vi "Teleop.vi"(10 "Match Info":T1={"Autonomous Elapsed Seconds"=0.0, "TeleOp Elapsed Seconds"=0.0, "Disabled Elapsed Seconds"=0.0, "Visited Autonomous"=FALSE, "Visited TeleOp"=FALSE, "Visited Disabled"=FALSE, "Autonomous Settings"={"Autonomous Style"=enum."Independent", "VI Refnum"=refnum}}, 11 "Call Context":T2) -> ()   [LabVIEW 2015]
doc: "This VI is called for each TeleOp packet received from the DS where the robot is not disabled. It is often used to read from the joysticks and update I/O or to update setpoints for timed control loops. It should complete and return within 20 milliseconds or it may miss DS packets."
uses:
  <vilib>/Rock Robotics/WPI/DriverStation/WPI_DriverStationDerivedRobotMode.ctl
  <vilib>/Rock Robotics/WPI/DriverStation/WPI_DriverStationMatch Info.ctl
  Robot Global Data.vi
  <vilib>/Rock Robotics/Network Tables/SD Write Number.vi
  <vilib>/Rock Robotics/WPI/Solenoid/Deprecated/WPI_SolenoidSetBool.vi
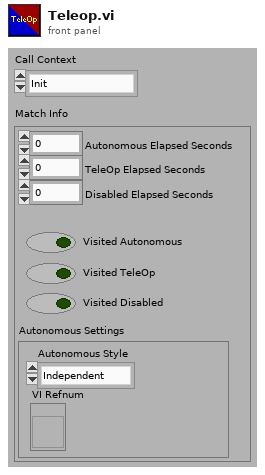
[diagram p1: front panel]
types:
  T1 = typedef "WPI_DriverStationMatch Info.ctl" = cluster{"Autonomous Elapsed Seconds":dbl, "TeleOp Elapsed Seconds":dbl, "Disabled Elapsed Seconds":dbl, "Visited Autonomous":bool, "Visited TeleOp":bool, "Visited Disabled":bool, "Autonomous Settings":cluster{"Autonomous Style":enum16{"Iterative", "Independent"}, "VI Refnum":refnum<vi>}}
  T2 = typedef "WPI_DriverStationDerivedRobotMode.ctl" = enum16{"Init", "Execute", "Stop"}
  T3 = typedef "WPI_MotorControlDeviceRef.ctl" = cluster{"DeviceStatus":errorcluster, "Type":T4, "PWM":cluster{"PWM Channel":T5, "DeadBand":T6}, "CAN":cluster{"Device Number":u8, "Control Mode":T7, "Semaphore":T8, "Max Vout":dbl, "TalonSRX Control Mode":T9}, "Invert":bool}
  T4 = typedef "WPI_MotorControlType.ctl" = enum16{"PWM", "CAN", "CANTalonSRX"}
  T5 = typedef "FPGA_DIOPWMChannel.ctl" = enum8{"PWM 0", "PWM 1", "PWM 2", "PWM 3", "PWM 4", "PWM 5", "PWM 6", "PWM 7", "PWM 8", "PWM 9", "PWM MXP 0", "PWM MXP 1", "PWM MXP 2", "PWM MXP 3", "PWM MXP 4", "PWM MXP 5", "PWM MXP 6", "PWM MXP 7", "PWM MXP 8", "PWM MXP 9", "Invalid"}
  T6 = typedef "WPI_PWMDeadband.ctl" = cluster{"Name":string, "maxPositivePwm":i32, "minPositivePwm":i32, "centerPwm":i32, "maxNegativePwm":i32, "minNegativePwm":i32, "angularRange":u16}
  T7 = typedef "WPI_CANJaguar_ControlMode.ctl" = enum8{"Percent VBus", "Current", "Speed", "Position", "Voltage"}
  T8 = typedef "Semaphore RefNum" = refnum<k1>
  T9 = typedef "WPI_CANTalonSRX_APIControlMode.ctl" = enum8{"Percent VBus", "Speed", "Position", "Slave", "Unchanged / Invalid", "Voltage Compensation", "Current", "Motion Profile"}
  T10 = typedef "WPI_CANTalonSRX_GlobalStatus.ctl" = cluster{"Applied Throttle":dbl, "Module Enabled":bool, "CAN Error":errorcluster, "Closed Loop Error":dbl, "Forward Limit Switch Closed":bool, "Reverse Limit Switch Closed":bool, "Sensor Position":dbl, "Sensor Velocity":dbl, "Current":dbl, "Sticky Fault - Over Temp":bool, "Sticky Fault - Under Voltage":bool, "Sticky Fault - Forward Limit":bool, "Sticky Fault - Reverse Limit":bool, "Sticky Fault - Forward Soft Limit":bool, "Sticky Fault - Reverse Soft Limit":bool, "Brake is Enabled":bool, "Encoder Position":dbl, "Encoder Velocity":dbl, "Encoder Index Count":dbl, "Encoder A Pin State":bool, "Encoder B Pin State":bool, "Encoder Index Pin State":bool, "Analog In":dbl, "Analog In Velocity":dbl, "Temperature (C)":dbl, "Battery Voltage":dbl, "Control 5 Is Supported":bool, "Current Profile Slot Select":dbl, "Pos Div 8":bool, "Vel Div 4":bool, "Pulse Width Position":i32, "Pulse Width Velocity":i32, "Pulse Width Rise To Rise (us)":i32, "Pulse Width Rise To Fall (us)":i32, "Mot Prof Active Is Under Run":bool, "Mot Prof Active Has Under Run":bool, "Mot Prof Active Is Last":bool, "Mot Prof Active Velocity Only":bool, "Mot Prof Active Is Valid":bool, "Mot Prof Buffer Is Full":bool, "Mot Prof Active Profile Slot Select":i32, "Mot Prof NextID":i32, "Mot Prof Count":i32, "Mot Prof Active Velocity":dbl, "Mot Prof Active Position":dbl, "Mot Prof Output Enable":i32}
  T11 = typedef "WPI_SolenoidDevRef.ctl" = cluster{"DevStatus":errorcluster, "Pneumatics Control Module":u8, "Forward Solenoid Channel":T12, "Reverse Solenoid Channel":T12}
  T12 = typedef "WPI_SolenoidChannel.ctl" = enum8{"Solenoid 0", "Solenoid 1", "Solenoid 2", "Solenoid 3", "Solenoid 4", "Solenoid 5", "Solenoid 6", "Solenoid 7", "Invalid"}
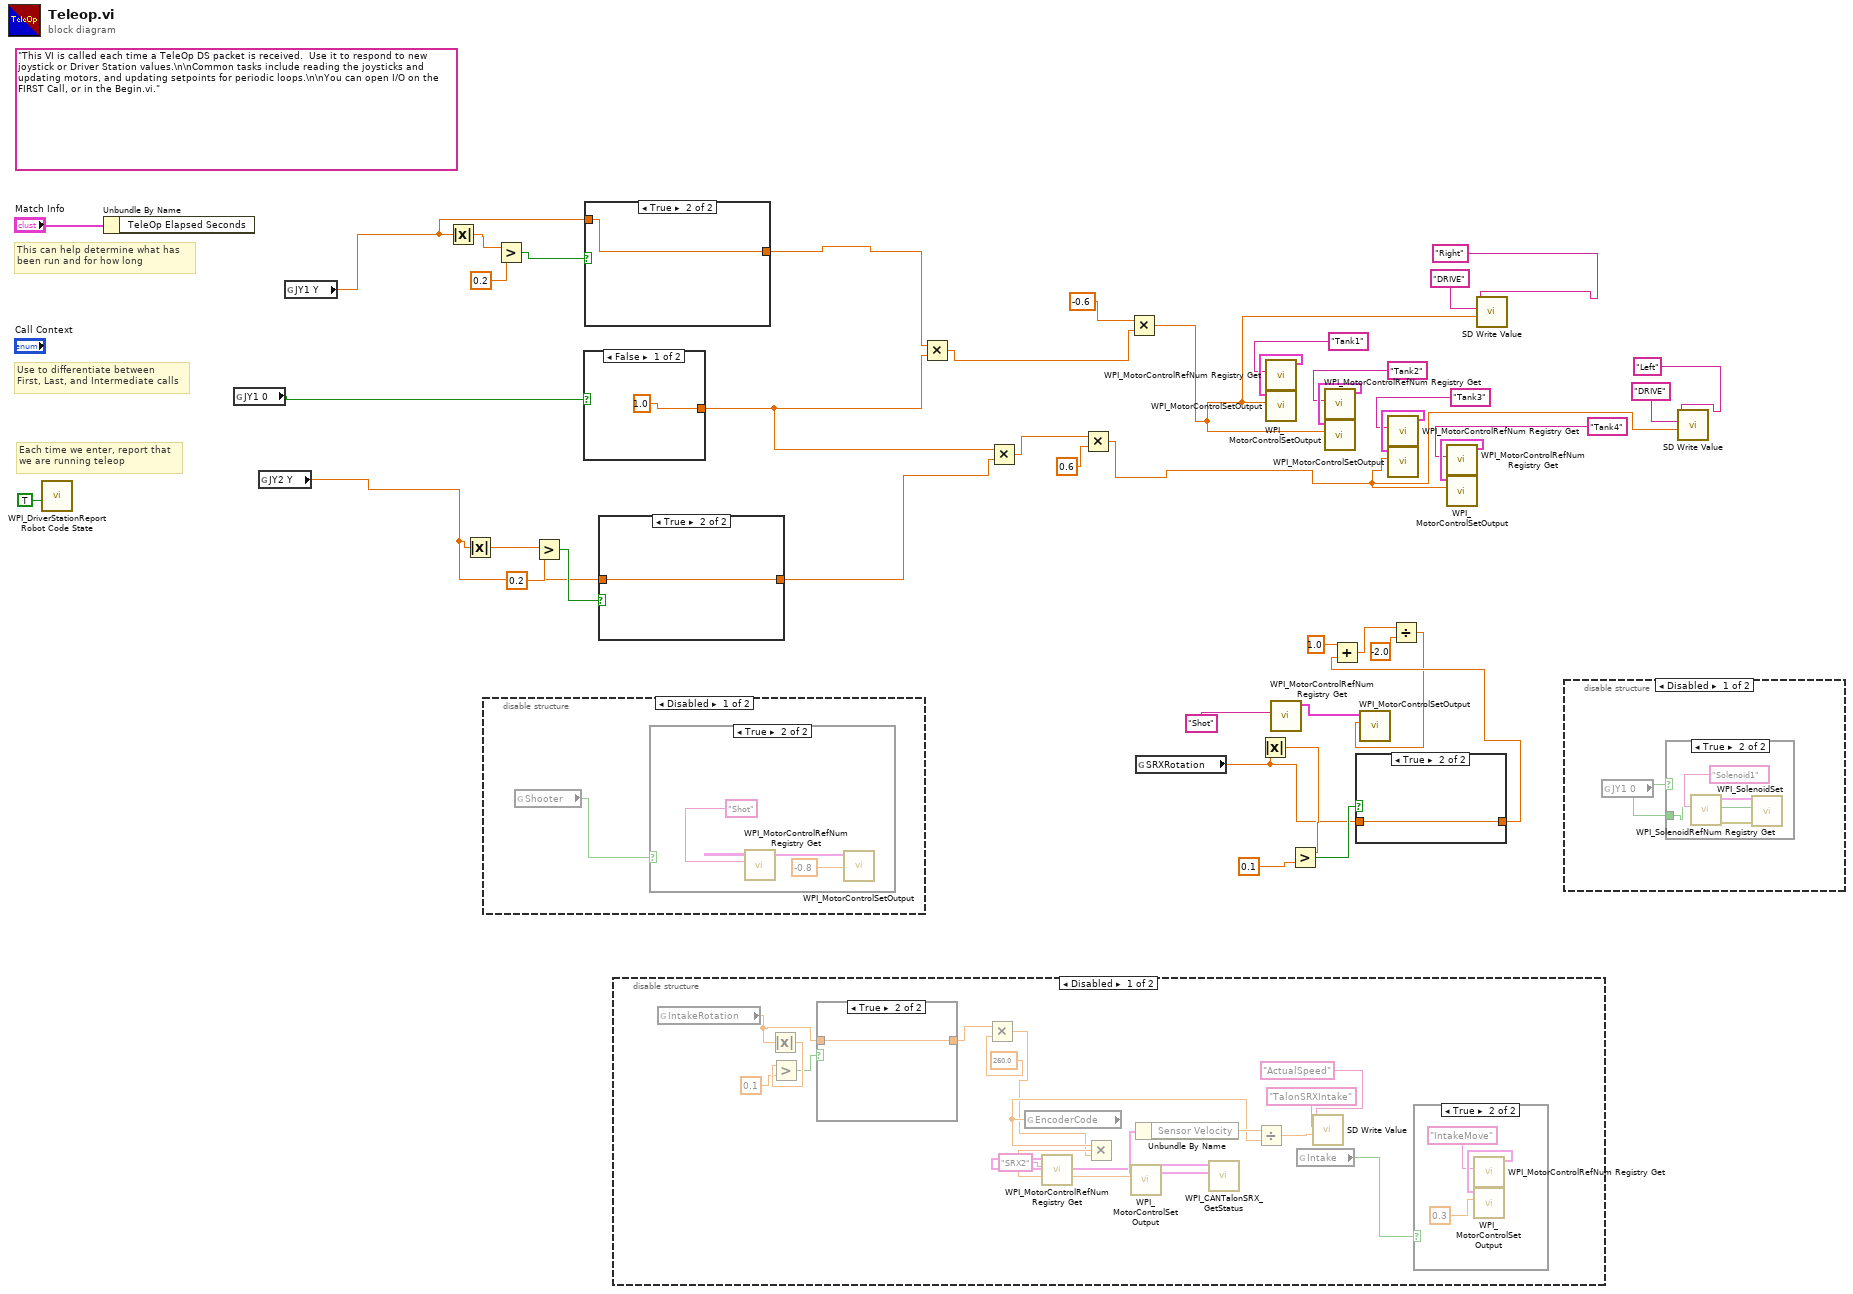
[diagram p0: block diagram]
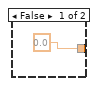
[diagram p6: hidden frame]
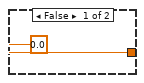
[diagram p9: hidden frame]
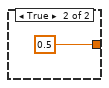
[diagram p10: hidden frame]
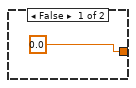
[diagram p11: hidden frame]
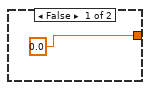
[diagram p12: hidden frame]
diagram:
  (unwired) "This VI is called each time a TeleOp DS packet is received.  Use it to respond to new joystick or Driver Station values.\n\nCommon tasks include reading the joysticks and updating motors, and updating setpoints for periodic loops.\n\nYou can open I/O on the FIRST Call, or in the Begin.vi."
  # "Each time we enter, report that\nwe are running teleop"
  # "Use to differentiate between\nFirst, Last, and Intermediate calls"
  # "This can help determine what has\nbeen run and for how long"
  n1 = call <vilib>:"WPI_DriverStationReport Robot Code State.vi"("TeleOp"=TRUE ("Autonomous")) -> ()  [unwired: 10 in, 1 out]
  n2 = Unbundle By Name("Match Info") -> ()  [unwired: 1 out]
  n3 = global read "Robot Global Data.vi" "JY1 0"() -> (w29:bool)
  n4 = global read "Robot Global Data.vi" "JY2 Y"() -> (w30:dbl)
  n5 = global read "Robot Global Data.vi" "JY1 Y"() -> (w31:dbl)
  n6 = Absolute Value(x=w31) -> (abs(x)=w34:dbl)
  n7 = Absolute Value(x=w30) -> (abs(x)=w33:dbl)
  n8 = disable-structure shown="Disabled" {
    frame Disabled {
      n9 = global read "Robot Global Data.vi" "Shooter"() -> (w44:bool)
      n10 = case shown="True" w44 {
        frame False {
        }
        frame True {
          n11 = call <vilib>:"WPI_MotorControlRefNum Registry Get.vi"("refnum name"="Shot") -> ("MotorControlDevRef"=w47:T3)  [unwired: 9 in, 1 out]
          n12 = call <vilib>:"WPI_MotorControlSetOutput.vi"("Output"=-0.8, "MotorControlDevRef"=w47) -> ()  [unwired: 7 in, 3 out]
        }
      }
    }
    frame Enabled {
    }
  }
  n13 = Greater?(x=w34, y=0.2) -> (0:w41:bool)
  n14 = Greater?(x=w33, y=0.2) -> (0:w39:bool)
  n15 = case shown="False" w29 {
    tunnel: [1.0 0.5] -> w37
    frame False {
    }
    frame True {
    }
  }
  n16 = case shown="True" w41 {
    tunnel: [0.0 w51] -> w13
    tunnel: w31 -> [_ w51]
    frame False {
    }
    frame True {
    }
  }
  n17 = case shown="True" w39 {
    tunnel: [0.0 w53] -> w14
    tunnel: w30 -> [_ _]
    tunnel: w30 -> [_ w53]
    frame False {
    }
    frame True {
    }
  }
  n18 = disable-structure shown="Disabled" {
    frame Disabled {
      n19 = global read "Robot Global Data.vi" "IntakeRotation"() -> (w67:dbl)
      n20 = Absolute Value(x=w67) -> (abs(x)=w70:dbl)
      n21 = Greater?(x=w70, y=0.1) -> (0:w68:bool)
      n22 = case shown="True" w68 {
        tunnel: w67 -> [_ w73]
        tunnel: [0.0 w73] -> w57
        frame False {
        }
        frame True {
        }
      }
      n23 = Multiply(x=w57, y=260.0) -> (x*y=w54:dbl)
      n24 = global read "Robot Global Data.vi" "EncoderCode"() -> (w62:dbl)
      n25 = call <vilib>:"WPI_MotorControlRefNum Registry Get.vi"("refnum name"="SRX2") -> ("MotorControlDevRef"=w60:T3)  [unwired: 9 in, 1 out]
      n26 = Multiply(x=w62, y=w54) -> (x*y=w63:dbl)
      n27 = call <vilib>:"WPI_MotorControlSetOutput.vi"("Output"=w63, "MotorControlDevRef"=w60) -> ("MotorControlDevRef"=w66:T3)  [unwired: 7 in, 2 out]
      n28 = call <vilib>:"WPI_CANTalonSRX_GetStatus.vi"("CAN Talon SRX Ref"=w66) -> ("Talon SRX Status"=w65:T10)  [unwired: 8 in, 2 out]
      n29 = Unbundle By Name(w65) -> ("Sensor Velocity"=w64:dbl)
      n30 = Divide(x=w64, y=w62) -> (x/y=w59:dbl)
      n31 = global read "Robot Global Data.vi" "Intake"() -> (w71:bool)
      n32 = call-poly <vilib>:"SD Write Value.vi"("Numeric"=w59, "Table Prefix"="TalonSRXIntake", "Name"="ActualSpeed") -> ()  [unwired: 7 in, 2 out]
      n33 = case shown="True" w71 {
        frame False {
        }
        frame True {
          n34 = call <vilib>:"WPI_MotorControlRefNum Registry Get.vi"("refnum name"="IntakeMove") -> ("MotorControlDevRef"=w76:T3)  [unwired: 9 in, 1 out]
          n35 = call <vilib>:"WPI_MotorControlSetOutput.vi"("Output"=0.3, "MotorControlDevRef"=w76) -> ()  [unwired: 7 in, 3 out]
        }
      }
    }
    frame Enabled {
    }
  }
  n36 = Multiply(x=w13, y=w37) -> (x*y=w12:dbl)
  n37 = Multiply(x=w37, y=w14) -> (x*y=w35:dbl)
  n38 = Multiply(x=w35, y=0.6) -> (x*y=w16:dbl)
  n39 = Multiply(x=-0.6, y=w12) -> (x*y=w15:dbl)
  n40 = global read "Robot Global Data.vi" "SRXRotation"() -> (w7:dbl)
  n41 = Absolute Value(x=w7) -> (abs(x)=w10:dbl)
  n42 = call <vilib>:"WPI_MotorControlRefNum Registry Get.vi"("refnum name"="Tank1") -> ("MotorControlDevRef"=w28:T3)  [unwired: 9 in, 1 out]
  n43 = call <vilib>:"WPI_MotorControlSetOutput.vi"("Output"=w15, "MotorControlDevRef"=w28) -> ()  [unwired: 7 in, 3 out]
  n44 = call <vilib>:"WPI_MotorControlRefNum Registry Get.vi"("refnum name"="Shot") -> ("MotorControlDevRef"=w6:T3)  [unwired: 9 in, 1 out]
  n45 = Greater?(x=w10, y=0.1) -> (0:w8:bool)
  n46 = call <vilib>:"WPI_MotorControlRefNum Registry Get.vi"("refnum name"="Tank2") -> ("MotorControlDevRef"=w26:T3)  [unwired: 9 in, 1 out]
  n47 = call <vilib>:"WPI_MotorControlSetOutput.vi"("Output"=w15, "MotorControlDevRef"=w26) -> ()  [unwired: 7 in, 3 out]
  n48 = case shown="True" w8 {
    tunnel: [0.0 w78] -> w4
    tunnel: w7 -> [_ w78]
    frame False {
    }
    frame True {
    }
  }
  n49 = Add(x=1.0, y=w4) -> (x+y=w2:dbl)
  n50 = call <vilib>:"WPI_MotorControlRefNum Registry Get.vi"("refnum name"="Tank3") -> ("MotorControlDevRef"=w24:T3)  [unwired: 9 in, 1 out]
  n51 = call <vilib>:"WPI_MotorControlSetOutput.vi"("Output"=w16, "MotorControlDevRef"=w24) -> ()  [unwired: 7 in, 3 out]
  n52 = Divide(x=w2, y=-2.0) -> (x/y=w1:dbl)
  n53 = call <vilib>:"WPI_MotorControlSetOutput.vi"("Output"=w1, "MotorControlDevRef"=w6) -> ()  [unwired: 7 in, 3 out]
  n54 = call <vilib>:"WPI_MotorControlRefNum Registry Get.vi"("refnum name"="Tank4") -> ("MotorControlDevRef"=w22:T3)  [unwired: 9 in, 1 out]
  n55 = call <vilib>:"WPI_MotorControlSetOutput.vi"("Output"=w16, "MotorControlDevRef"=w22) -> ()  [unwired: 7 in, 3 out]
  n56 = call-poly <vilib>:"SD Write Value.vi"("Numeric"=w15, "Table Prefix"="DRIVE", "Name"="Right") -> ()  [unwired: 7 in, 2 out]
  n57 = disable-structure shown="Disabled" {
    frame Disabled {
      n58 = global read "Robot Global Data.vi" "JY1 0"() -> (w79:bool)
      n59 = case shown="True" w79 {
        tunnel: w79 -> [_ w80]
        frame False {
        }
        frame True {
          n60 = call <vilib>:"WPI_SolenoidRefNum Registry Get.vi"("refnum name"="Solenoid1") -> ("error out"=w82:errorcluster, "SolenoidDevRef"=w83:T11)  [unwired: 9 in]
          n61 = call-poly <vilib>:"WPI_SolenoidSet.vi"("error in (no error)"=w82, "Value"=w80, "SolenoidDevRef"=w83) -> ()  [unwired: 9 out]
        }
      }
    }
    frame Enabled {
    }
  }
  n62 = call-poly <vilib>:"SD Write Value.vi"("Numeric"=w16, "Table Prefix"="DRIVE", "Name"="Left") -> ()  [unwired: 7 in, 2 out]
